vi "FaceDistancesToCurrenArray.vi"(8 "error in (no error)":errorcluster, 11 "FaceDistances in":refnum<k24>) -> (0 "error out":errorcluster, 2 "CurrentArray":dbl[](array[numeric]), 3 "FaceDistances out":refnum<k24>)   [LabVIEW 2020, in "FaceRecognitionDotNet.lvlib" / "FaceRecognition.lvclass"]
uses:
  FaceRecognition.lvclass
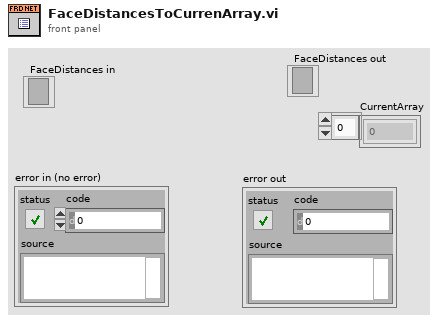
[diagram p1: front panel]
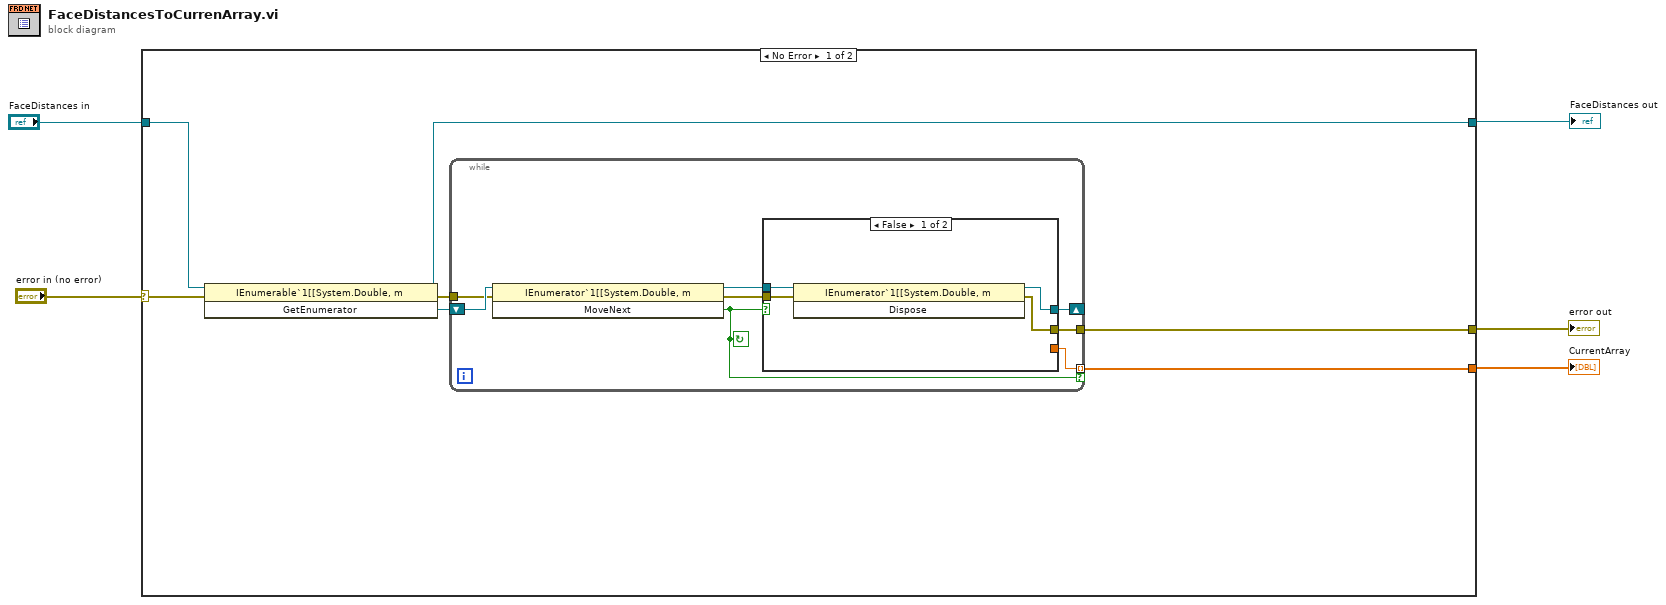
[diagram p0: block diagram]
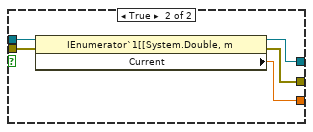
[diagram p2: hidden frame]
diagram:
  n1 = case shown="No Error" "error in (no error)" {
    selector: "error in (no error)" -> [w6 w30]
    tunnel: [w10 _] -> w5
    tunnel: [w9 w31] -> w4
    tunnel: [w8 w30] -> w3
    tunnel: "FaceDistances in" -> [w7 w31]
    frame No Error {
      n2 = invoke class="IEnumerable`1[[System.Double, m" method="GetEnumerator"(reference=w7, error in=w6) -> (reference out=w9:refnum<k24>, error out=w11:errorcluster, "GetEnumerator"=w12:refnum<k24>)  [unwired: 1 in]
      n3 = while {
        shift-right: [w17] -> _
        shift-left: w12 -> [w20]
        tunnel: w11 -> [w16]
        tunnel: [w15] -> w8
        tunnel: [w14] -> w10 mode=indexing if=w13
        stop <- w13 continue-if-true
        n4 = invoke class="IEnumerator`1[[System.Double, m" method="MoveNext"(reference=w20, error in=w16) -> (reference out=w19:refnum<k24>, error out=w18:errorcluster, "MoveNext"=w13:bool)  [unwired: 1 in]
        n5 = case shown="False" w13 {
          tunnel: w19 -> [w24 w29]
          tunnel: w18 -> [w22 w28]
          tunnel: [w23 w27] -> w17
          tunnel: [w21 w26] -> w15
          tunnel: [_ w25] -> w14
          frame False {
            n6 = invoke class="IEnumerator`1[[System.Double, m" method="Dispose"(reference=w24, error in=w22) -> (reference out=w23:refnum<k24>, error out=w21:errorcluster)  [unwired: 1 in, 1 out]
          }
          frame True {
            n7 = property class="IEnumerator`1[[System.Double, m"(reference=w29, error in=w28) -> (reference out=w27:refnum<k24>, error out=w26:errorcluster, "Current"=w25:dbl)
          }
        }
      }
    }
    frame Error {
    }
  }
  "FaceDistances out" <- w4
  "CurrentArray" <- w5
  "error out" <- w3
